vi "SS Test Seq Description.vi"(11 "Test Seq":T2[](array[typedef])=[{"Seq#"=1.0, "Draw"=35.0, "Cycles"=4, "Mode Read"=enum."Hybrid"}, {"Seq#"=2.0, "Draw"=15.0, "Cycles"=9, "Mode Read"=enum."Hybrid"}, {"Seq#"=3.0, "Draw"=35.0, "Cycles"=2, "Mode Read"=enum."eHeat"}, {"Seq#"=4.0, "Draw"=15.0, "Cycles"=5, "Mode Read"=enum."eHeat"}, {"Seq#"=5.0, "Draw"=35.0, "Cycles"=2, "Mode Read"=enum."StdElectric"}, {"Seq#"=6.0, "Draw"=15.0, "Cycles"=5, "Mode Read"=enum."StdElectric"}, {"Seq#"=7.0, "Draw"=35.0, "Cycles"=2, "Mode Read"=enum."Hybrid"}, {"Seq#"=8.0, "Draw"=15.0, "Cycles"=5, "Mode Read"=enum."Hybrid"}]) -> (3 "Out Description":string[](array[string]))   [LabVIEW 2011]
uses:
  HEWH PRAT/PRAT Test.ctl
  Hybrid Water Heater/GEA2/HEWH_Mode.ctl
panel:
  out "Mode Read":T1=enum."HighDemand"
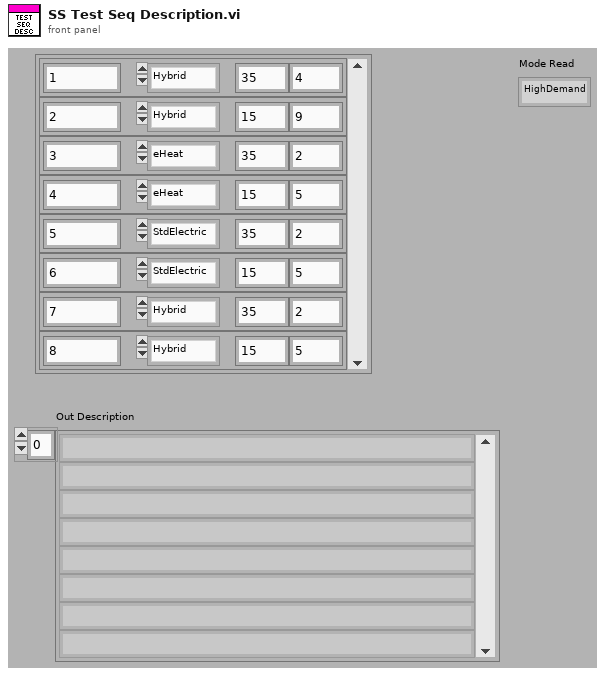
[diagram p1: front panel]
types:
  T1 = typedef "HEWH_Mode.ctl" = enum16{"Hybrid", "StdElectric", "eHeat", "HighDemand", "Vacation"}
  T2 = typedef "PRAT Test.ctl" = cluster{"Seq#":dbl, "Draw":dbl, "Cycles":i32, "Mode Read":T1}
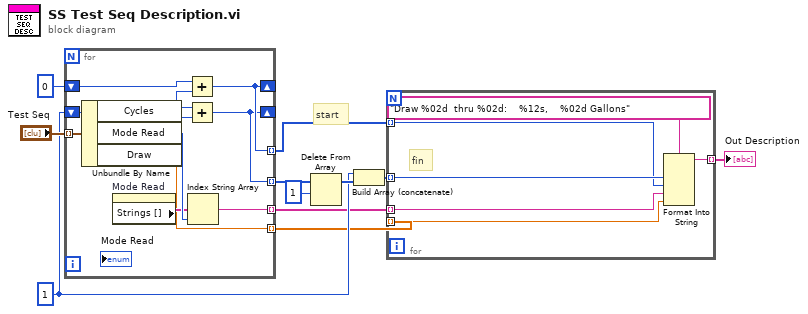
[diagram p0: block diagram]
diagram:
  w6 = 1
  # "fin"
  # "start"
  n1 = for {
    tunnel: "Test Seq" -> [w21] mode=indexing
    shift-right: [w19] -> _
    shift-left: 0 -> [w20]
    tunnel: [w19] -> w4 mode=indexing
    shift-right: [w16] -> _
    shift-left: w6 -> [w17]
    tunnel: [w16] -> w9 mode=indexing
    tunnel: [w13] -> w2 mode=indexing
    tunnel: [w12] -> w1 mode=indexing
    n2 = Unbundle By Name(w21) -> ("Cycles"=w18:i32, "Mode Read"=w15:T1, "Draw"=w12:dbl)
    n3 = property on="Mode Read" class="Enum (strict)"() -> ("Strings []"=w14:string[])  [unwired: 2 in, 2 out]
    n4 = Add(x=w20, y=w18) -> (x+y=w19:i32)
    n5 = Add(x=w17, y=w18) -> (x+y=w16:i32)
    n6 = Index String Array(1:w15, 2:w14) -> (0:w13:string)  [unwired: 1 in]
  }
  n7 = Delete From Array(array=w9, length=1) -> (array with subset deleted=w7:i32[])  [unwired: 1 in, 1 out]
  n8 = Build Array (concatenate)(w6, w7) -> (w5:i32[])
  n9 = for {
    tunnel: w5 -> [w27] mode=indexing
    tunnel: w4 -> [w26] mode=indexing
    tunnel: [w25] -> w3 mode=indexing
    tunnel: w2 -> [w24] mode=indexing
    tunnel: w1 -> [w23] mode=indexing
    n10 = Format Into String(format string="Draw %02d  thru %02d:    %12s,    %02d Gallons", w27, w26, w24, w23) -> (resulting string=w25:string)  [unwired: 2 in, 1 out]
  }
  "Out Description" <- w3
